vi "Drive_self_test.vi"() -> ()   [LabVIEW 2017, in "labview-standard-library.lvlib"]
uses:
  labview-standard-library.lvlib
  Drive_test_states.ctl
panel:
  in  "Test reverse?":bool=TRUE
  out "Average encoder velocity":dbl
  out "Waveform Chart":dbl(graph)
  out "Final Encoder Value":dbl
  out "Power out 2":dbl(graph)
  out "Average current":dbl
  out "Power out":dbl format="%#_13g"
  in  "stop":bool
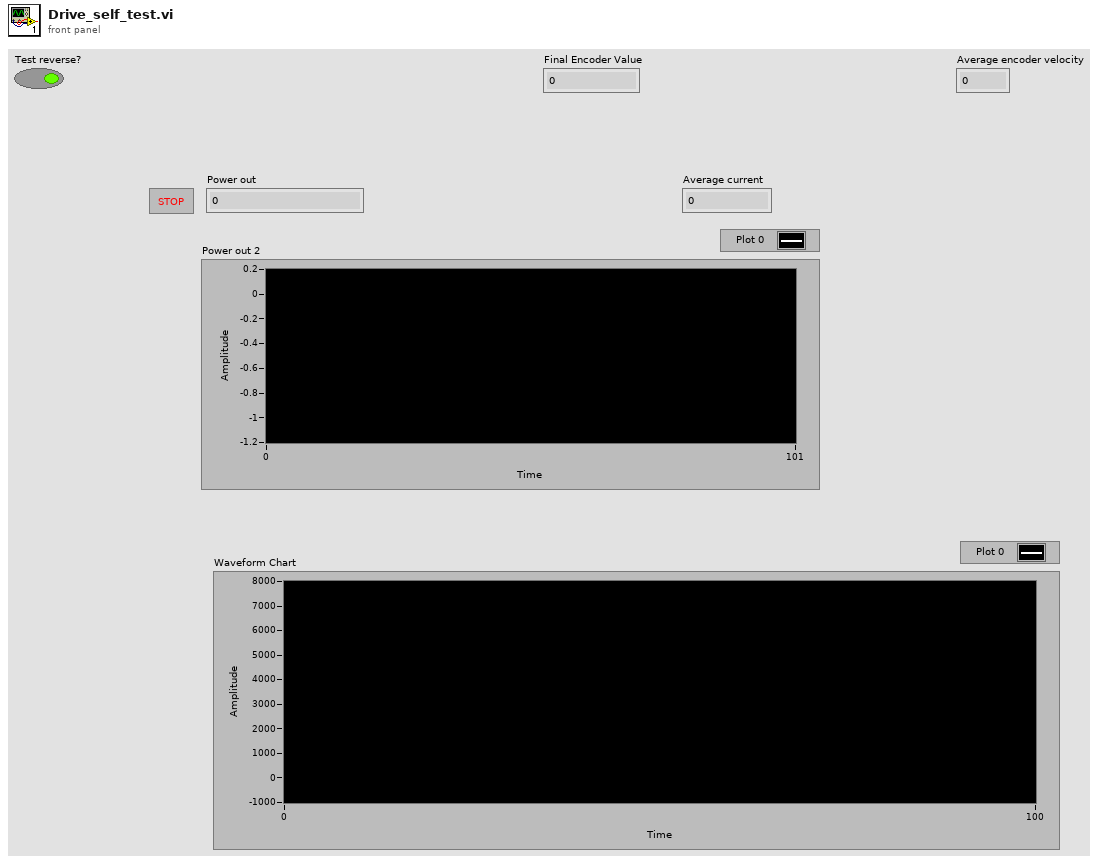
[diagram p1: front panel]
types:
  T1 = typedef "labview-standard-library.lvlib/Drive_test_states.ctl" = enum16{"Ramp Up", "Full Speed", "Ramp Down"}
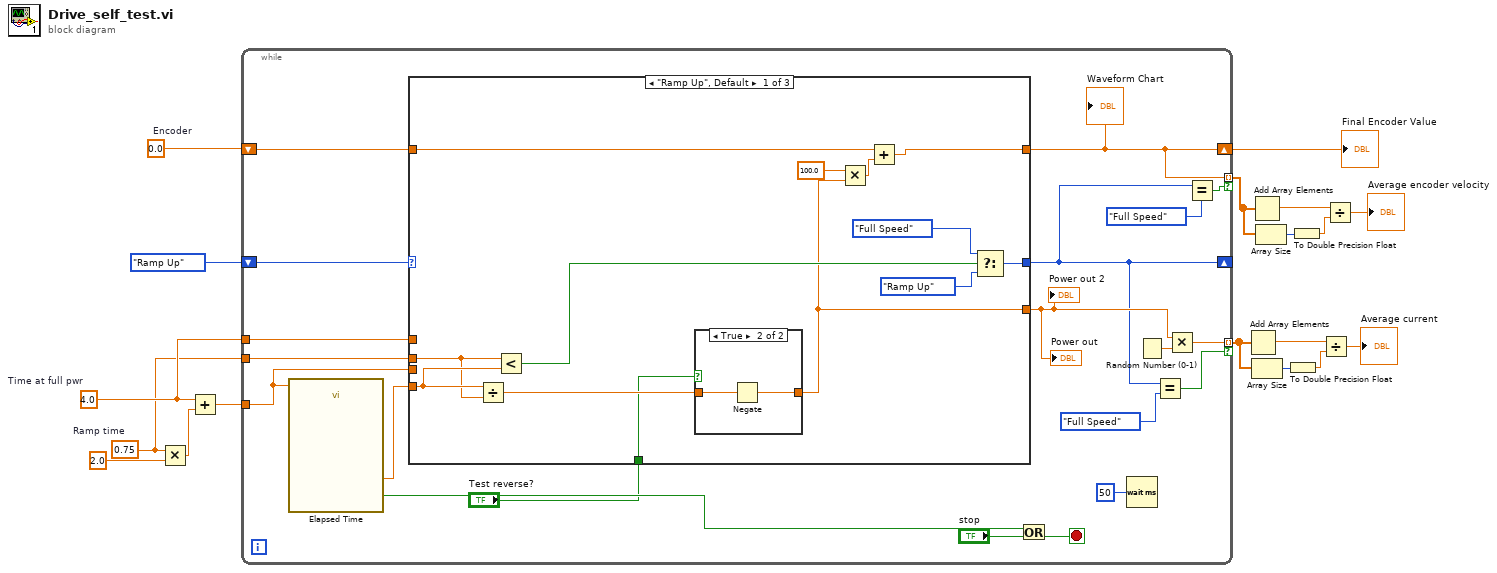
[diagram p0: block diagram]
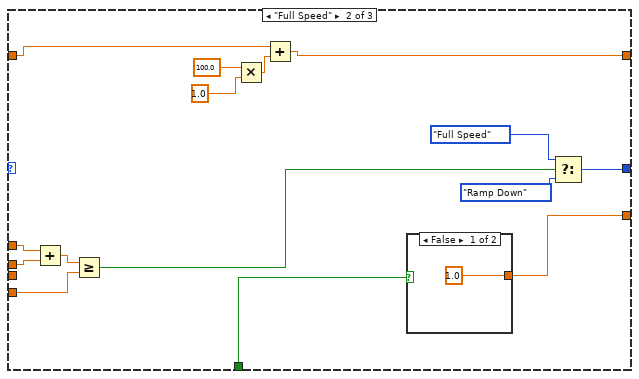
[diagram p3: hidden frame]
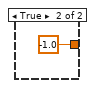
[diagram p4: hidden frame]
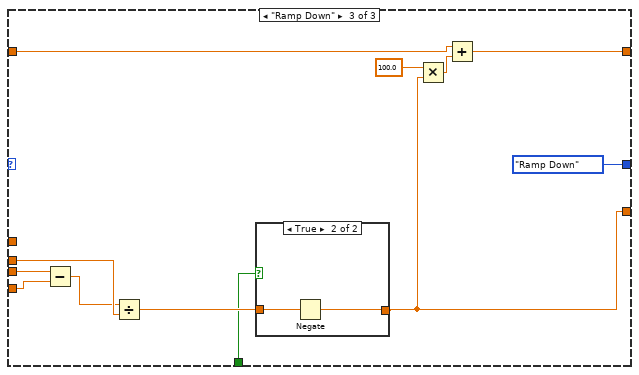
[diagram p5: hidden frame]
diagram:
  w7 = 0.0  # Encoder
  w13 = 0.75  # Ramp time
  w14 = 4.0  # Time at full pwr
  n1 = Multiply(x=w13, y=2.0) -> (x*y=w17:dbl)
  n2 = Add(x=w14, y=w17) -> (x+y=w16:dbl)
  n3 = while {
    tunnel: w16 -> [w30]
    shift-right: [w21] -> _
    shift-left: Drive_test_states."Ramp Up" -> [w33]
    tunnel: w14 -> [w32]
    tunnel: w13 -> [w31]
    tunnel: [w28] -> w12 mode=indexing if=w27
    shift-right: [w23] -> w6
    shift-left: w7 -> [w24]
    tunnel: [w23] -> w1 mode=indexing if=w20
    stop <- w36 stop-if-true
    n4 = call "Elapsed Time"("Time Target (s)"=w30) -> ("Elapsed Time (s)"=w34:dbl, "Time has Elapsed"=w35:bool)  [unwired: 11 in, 6 out]
    n5 = case shown="\"Ramp Up\", Default" w33 {
      tunnel: w34 -> [w47 w66 w81]
      tunnel: [w40 w61 w73] -> w25
      tunnel: [w49 w63 Drive_test_states."Ramp Down"] -> w21
      tunnel: w32 -> [_ w69 _]
      tunnel: w31 -> [w46 w68 w80]
      tunnel: w30 -> [_ _ w82]
      tunnel: w24 -> [w45 w58 w76]
      tunnel: [w42 w56 w75] -> w23
      tunnel: "Test reverse?" -> [w39 w55 w72]
      frame "Ramp Up", Default {
        n6 = Divide(x=w47, y=w46) -> (x/y=w41:dbl)
        n7 = Less?(x=w46, y=w47) -> (x < y?=w48:bool)
        n8 = case shown="True" w39 {
          tunnel: w41 -> [w52 w54]
          tunnel: [w52 w53] -> w40
          frame False {
          }
          frame True {
            n9 = Negate(x=w54) -> (-x=w53:dbl)
          }
        }
        n10 = Multiply(x=100.0, y=w40) -> (x*y=w44:dbl)
        n11 = Add(x=w45, y=w44) -> (x+y=w42:dbl)
        n12 = Select(t=Drive_test_states."Full Speed", s=w48, f=Drive_test_states."Ramp Up") -> (s? t:f=w49:T1)
      }
      frame "Full Speed" {
        n13 = Add(x=w69, y=w68) -> (x+y=w67:dbl)
        n14 = Greater Or Equal?(x=w67, y=w66) -> (x >= y?=w62:bool)
        n15 = Multiply(x=100.0, y=1.0) -> (x*y=w60:dbl)
        n16 = Add(x=w58, y=w60) -> (x+y=w56:dbl)
        n17 = case shown="False" w55 {
          tunnel: [1.0 -1.0] -> w61
          frame False {
          }
          frame True {
          }
        }
        n18 = Select(t=Drive_test_states."Full Speed", s=w62, f=Drive_test_states."Ramp Down") -> (s? t:f=w63:T1)
      }
      frame "Ramp Down" {
        n19 = Subtract(x=w82, y=w81) -> (x-y=w79:dbl)
        n20 = Divide(x=w79, y=w80) -> (x/y=w74:dbl)
        n21 = case shown="True" w72 {
          tunnel: [w84 w85] -> w73
          tunnel: w74 -> [w84 w86]
          frame False {
          }
          frame True {
            n22 = Negate(x=w86) -> (-x=w85:dbl)
          }
        }
        n23 = Multiply(x=100.0, y=w73) -> (x*y=w78:dbl)
        n24 = Add(x=w76, y=w78) -> (x+y=w75:dbl)
      }
    }
    "Power out" <- w25
    "Power out 2" <- w25
    "Waveform Chart" <- w23
    n25 = Or(x=w35, y="stop") -> (x .or. y?=w36:bool)
    n26 = Wait (ms)(milliseconds to wait=u32 50) -> ()  [unwired: 1 out]
    n27 = Random Number (0-1)() -> (number: 0 to 1=w29:dbl)
    n28 = Equal?(x=w21, y=Drive_test_states."Full Speed") -> (x = y?=w27:bool)
    n29 = Multiply(x=w25, y=w29) -> (x*y=w28:dbl)
    n30 = Equal?(x=w21, y=Drive_test_states."Full Speed") -> (x = y?=w20:bool)
  }
  "Final Encoder Value" <- w6
  n31 = Add Array Elements(numeric array=w12) -> (sum=w11:dbl)
  n32 = Add Array Elements(numeric array=w1) -> (sum=w3:dbl)
  n33 = Array Size(array=w12) -> (size(s)=w10:i32)
  n34 = Array Size(array=w1) -> (size(s)=w4:i32)
  n35 = To Double Precision Float(number=w10) -> (double precision float=w8:dbl)
  n36 = To Double Precision Float(number=w4) -> (double precision float=w5:dbl)
  n37 = Divide(x=w11, y=w8) -> (x/y=→"Average current":dbl)
  n38 = Divide(x=w3, y=w5) -> (x/y=→"Average encoder velocity":dbl)
